vi "Create Timing.vi"(8 "error in (no error)":errorcluster, 9 "Offset":u64, 10 "Decimation":u64=1, 11 "Priority":u64) -> (0 "error out":errorcluster, 3 "Timing":refnum<class "Timing.lvclass">)   [LabVIEW 2017, in "DSF Core.lvlib" / "Timing.lvclass"]
uses:
  Timing.lvclass
  Timing.lvclass/Timing.ctl
  Invalid Offset.vi
  Invalid Priority.vi
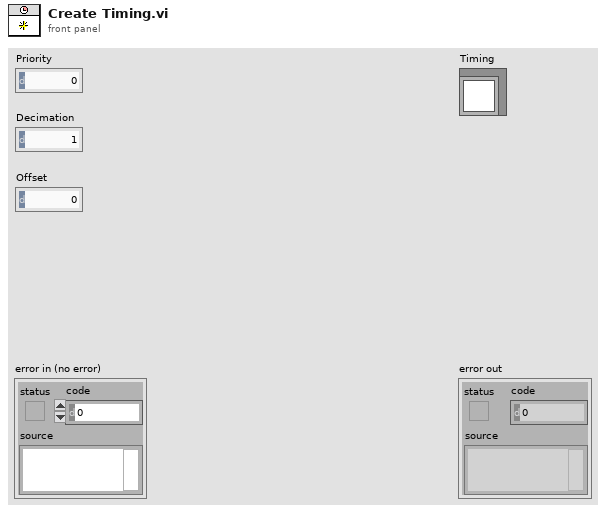
[diagram p1: front panel]
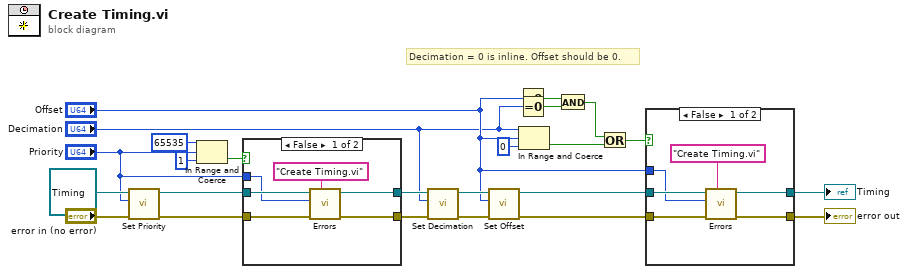
[diagram p0: block diagram]
diagram:
  # "Decimation = 0 is inline. Offset should be 0."
  n1 = call "Set Priority.vi"("Priority"="Priority", "Timing in"=refnum<class "Timing.lvclass"> refnum ("Timing")) -> ("Timing out"=w9:refnum<class "Timing.lvclass">)  [unwired: 9 in]
  n2 = In Range and Coerce(upper limit=u64 65535, x="Priority", lower limit=u64 1) -> (In Range?=w2:bool)  [unwired: 1 out]
  n3 = case shown="False" w2 {
    tunnel: w9 -> [w27 w29]
    tunnel: [w26 w29] -> w8
    tunnel: "error in (no error)" -> [w25 w28]
    tunnel: [w24 w28] -> w6
    tunnel: "Priority" -> [w22 _]
    frame False {
      n4 = call-poly "Errors.vi"("error source vi name"="Create Timing.vi", "error in (no error)"=w25, "priority"=w22, "Timing in"=w27) -> ("error out"=w24:errorcluster, "Timing out"=w26:refnum<class "Timing.lvclass">)  [unwired: 6 in]
    }
    frame True {
    }
  }
  n5 = call "Set Decimation.vi"("Decimation"="Decimation", "Timing in"=w8) -> ("Timing out"=w20:refnum<class "Timing.lvclass">)  [unwired: 9 in]
  n6 = call "Set Offset.vi"("Offset"="Offset", "Timing in"=w20) -> ("Timing out"=w18:refnum<class "Timing.lvclass">)  [unwired: 9 in]
  n7 = Equal To 0?(x="Offset") -> (x = 0?=w13:bool)
  n8 = Equal To 0?(x="Decimation") -> (x = 0?=w14:bool)
  n9 = In Range and Coerce(upper limit="Decimation", x="Offset", lower limit=u64 0) -> (In Range?=w12:bool)  [unwired: 1 out]
  n10 = And(x=w13, y=w14) -> (x .and. y?=w10:bool)
  n11 = Or(x=w10, y=w12) -> (x .or. y?=w11:bool)
  n12 = case shown="False" w11 {
    tunnel: w18 -> [w35 w37]
    tunnel: [w34 w37] -> w17
    tunnel: [w33 w36] -> w16
    tunnel: w6 -> [w32 w36]
    tunnel: "Offset" -> [w31 _]
    frame False {
      n13 = call-poly "Errors.vi"("error source vi name"="Create Timing.vi", "error in (no error)"=w32, "offset"=w31, "Timing in"=w35) -> ("error out"=w33:errorcluster, "Timing out"=w34:refnum<class "Timing.lvclass">)  [unwired: 6 in]
    }
    frame True {
    }
  }
  "error out" <- w16
  "Timing" <- w17
